vi "Set Edge Trigger.vi"(6 "Trigger Slope (0: Rising)":u16(ring) items=["Rising", "Falling", "Either"], 7 "Trigger Coupling (0 : DC)":u16(ring) items=["DC", "HF Reject", "LF Reject", "Noise Reject", "AC"], 8 "error in (no error)":errorcluster, 9 "Trigger Level (0.0 V)":dbl, 10 "Analog Channels":T1, 11 "DPO4104 in":refnum<class "DPO4104.lvclass">) -> (0 "error out":errorcluster, 3 "DPO4104 out":refnum<class "DPO4104.lvclass">)   [LabVIEW 2018, in "DPO4104.lvlib" / "DPO4104.lvclass"]
uses:
  DPO4104.lvclass
  PPLs/Oscilloscope/Parent/Oscilloscope.lvlibp/Custom Controls/Analog Channels.ctl
  <instrlib>/Tektronix DPO MSO 2000 4000 Series/Public/Configure/Configure Trigger (Edge).vi
  PPLs/Oscilloscope/Parent/Oscilloscope.lvlibp/Oscilloscope.lvclass
  <instrlib>/Tektronix DPO MSO 2000 4000 Series/Tektronix DPO MSO 2000 4000 Series.lvlib
  C:/Projects/LabVIEW/PPLs/Oscilloscope/Parent/Oscilloscope.lvlibp/Oscilloscope.lvclass
  PPLs/Oscilloscope/Parent/Oscilloscope.lvlibp
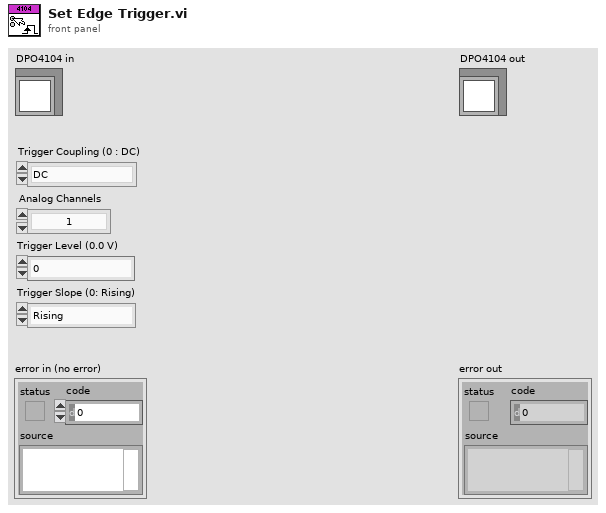
[diagram p1: front panel]
types:
  T1 = typedef "Oscilloscope.lvlibp/Analog Channels.ctl" = enum16{"1", "2", "3", "4", "5", "6", "7", "8", "9", "10", "11", "12", "13", "14", "15", "16"}
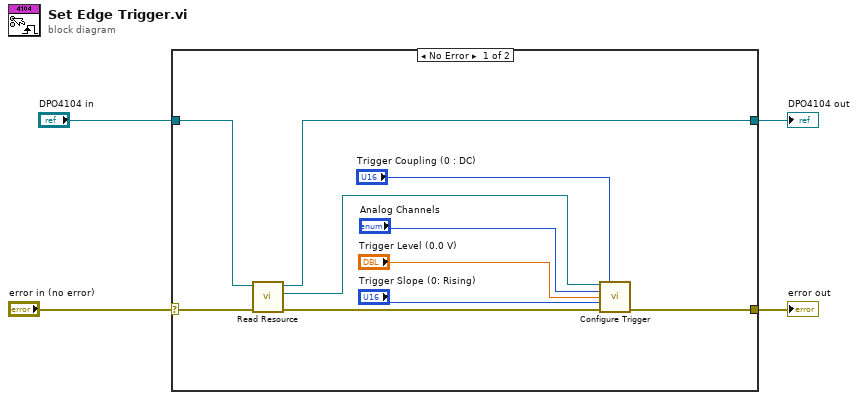
[diagram p0: block diagram]
diagram:
  n1 = case shown="No Error" "error in (no error)" {
    selector: "error in (no error)" -> [w14 w16]
    tunnel: [w9 w16] -> w3
    tunnel: "DPO4104 in" -> [w13 w15]
    tunnel: [w8 w15] -> w1
    frame No Error {
      n2 = call "Read Resource.vi"("error in (no error)"=w14, "Oscilloscope in"=w13) -> ("error out"=w12:errorcluster, "Resource"=w6:refnum<visa-resource-name>, "Oscilloscope out"=w8:refnum<class "DPO4104.lvclass">)  [unwired: 7 in]
      n3 = call-poly <instrlib>:"Configure Trigger.vi"("VISA resource name"=w6, "Trigger Coupling (0 : DC)"="Trigger Coupling (0 : DC)", "Trigger Source (0: Channel 1)"="Analog Channels", "Trigger Level (0.0 V)"="Trigger Level (0.0 V)", "Trigger Slope (0: Rising)"="Trigger Slope (0: Rising)", "error in (no error)"=w12) -> ("error out"=w9:errorcluster)  [unwired: 8 in, 1 out]
    }
    frame Error {
    }
  }
  "error out" <- w3
  "DPO4104 out" <- w1
